vi "Test Tree Structure.vi"() -> ()   [LabVIEW 2014]
uses:
  ERP-Manage Work Orders/ERP-ManageWorkOrders.lvclass
panel:
  in  "Discard?":bool
  out "Navigate Tree:Get Parent Item 2":string
  out "Col 2":i32
  out "Tag":string
  out "String":string
  out "Navigate Tree:Get Child 2":string
  out "Array 2":string[](array[string])
  out "Navigate Tree:Get Parent Item":string
  out "Active Cell:String":string
  out "All Tags":string[](array[string])
  out "Navigate Tree:Get Child":string
  in  "Stop Button":bool
  out "Array":T1(array[cluster])
  in  "Tree":string(tree)
  in  "Data IN":string[][](array[string])
  in  "Items":T1(array[cluster])
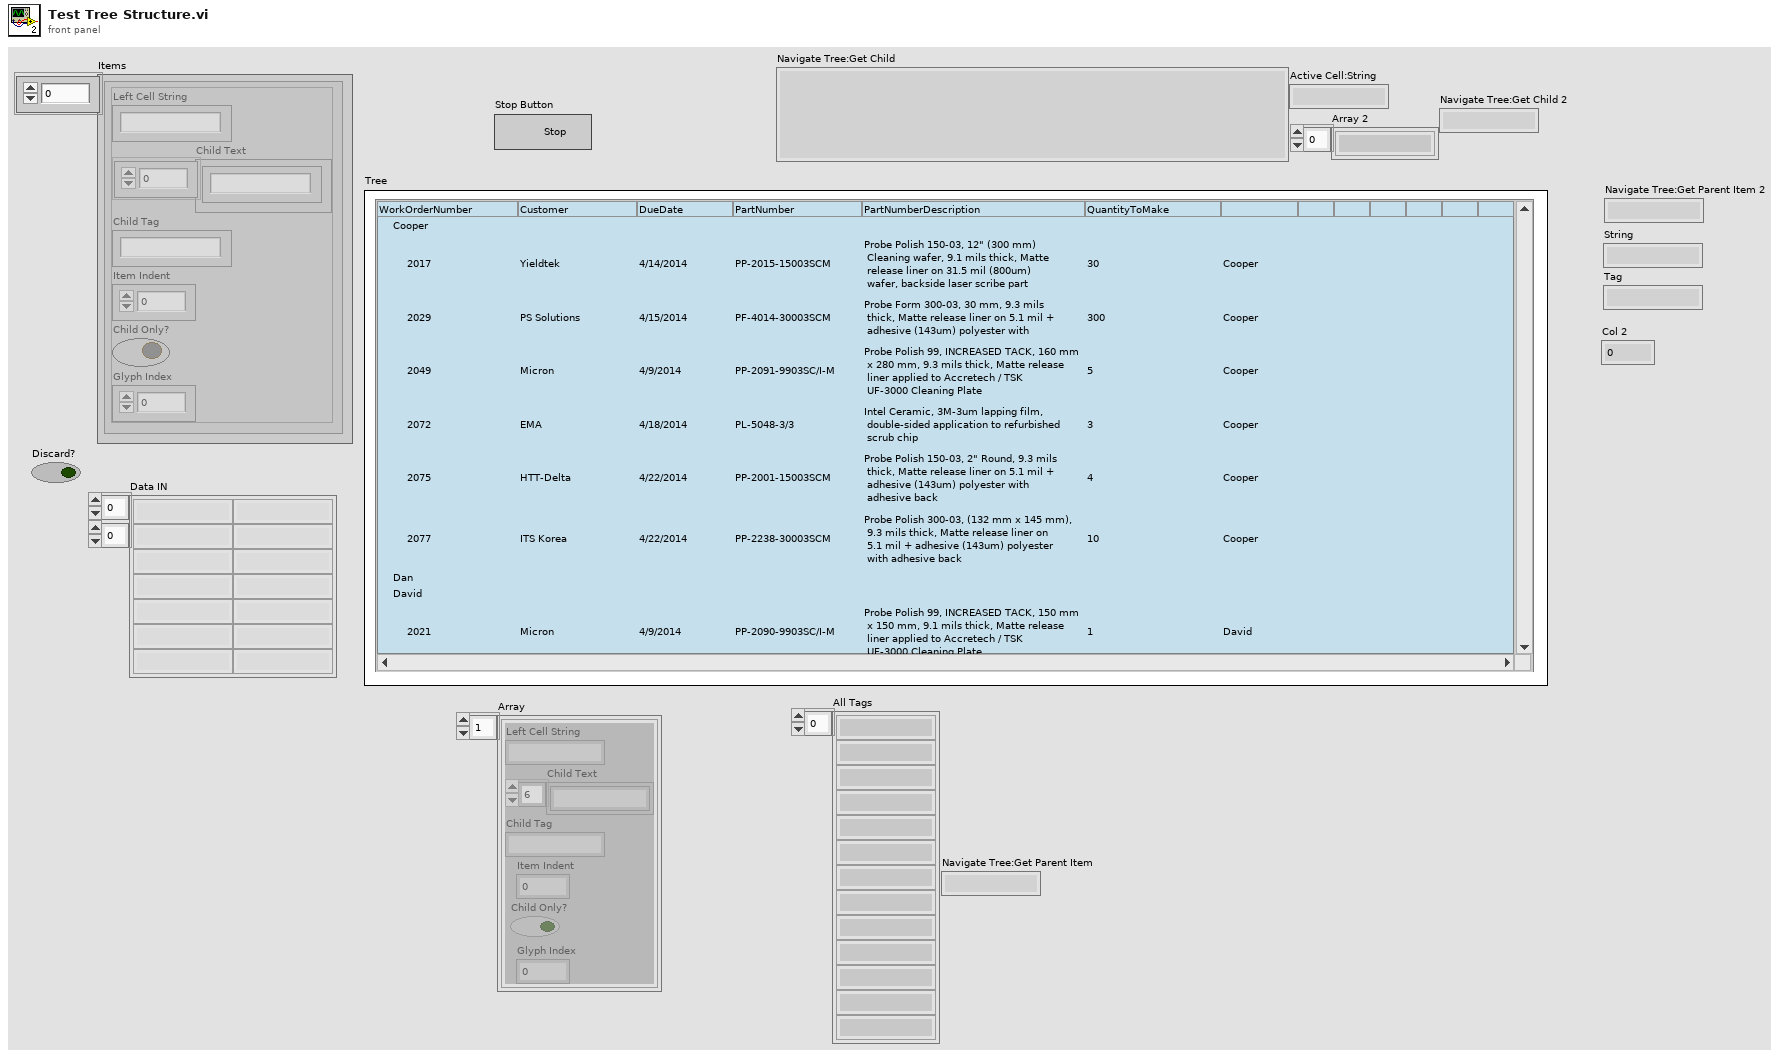
[diagram p1: front panel]
types:
  T1 = cluster{"Left Cell String":string, "Child Text":string[], "Child Tag":string, "Item Indent":i32, "Child Only?":bool, "Glyph Index":i32}[]
  T2 = cluster{"Left Cell String":string, "Child Text":string[], "Child Tag":string, "Item Indent":i32, "Child Only?":bool, "Glyph Index":i32}
  T3 = cluster{"data name":string, "drag data":variant}[]
  T4 = typedef "LVPoint32TypeDef.ctl" = cluster{"Horizontal":i32, "Vertical":i32}
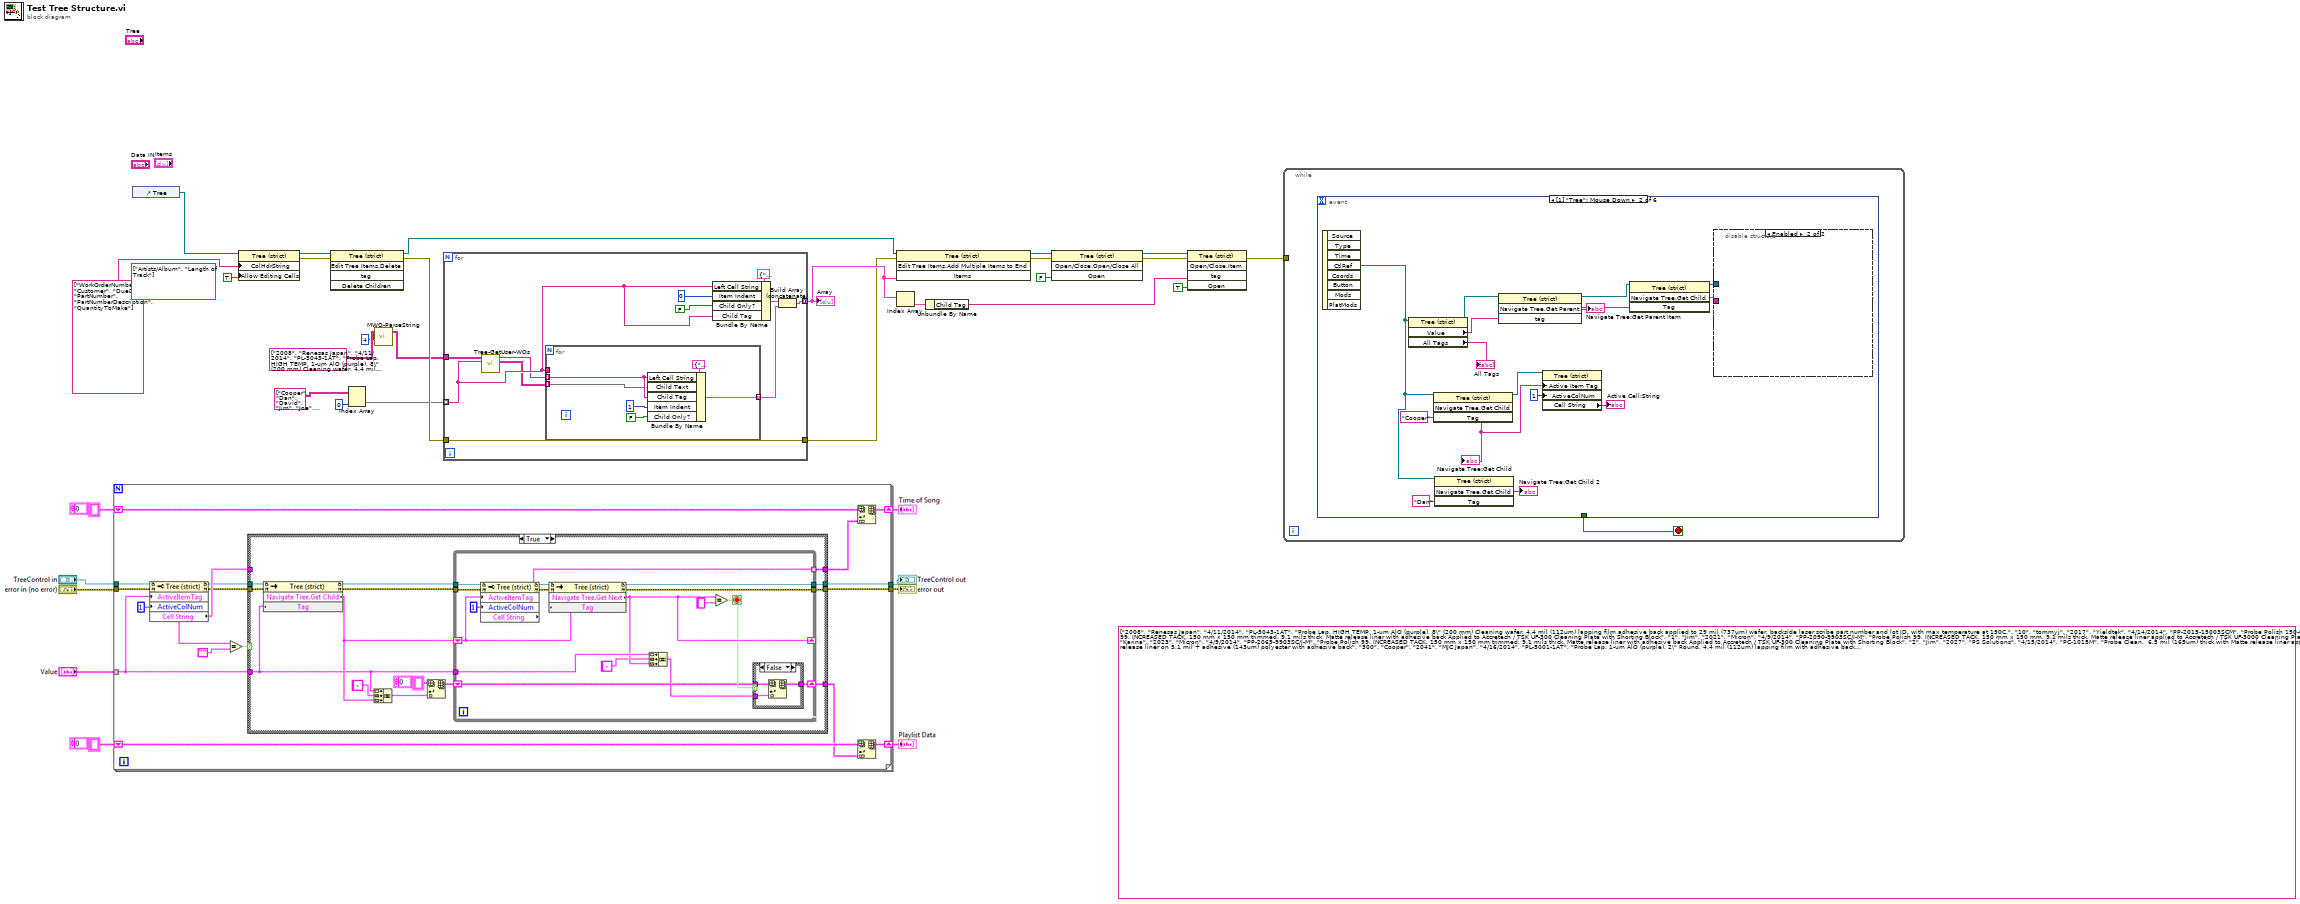
[diagram p0: block diagram]
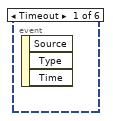
[diagram p2: hidden frame]
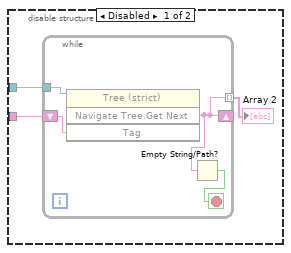
[diagram p3: hidden frame]
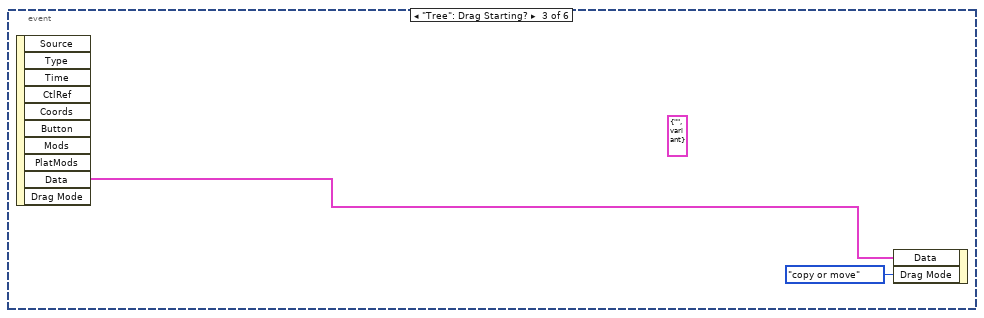
[diagram p4: hidden frame]
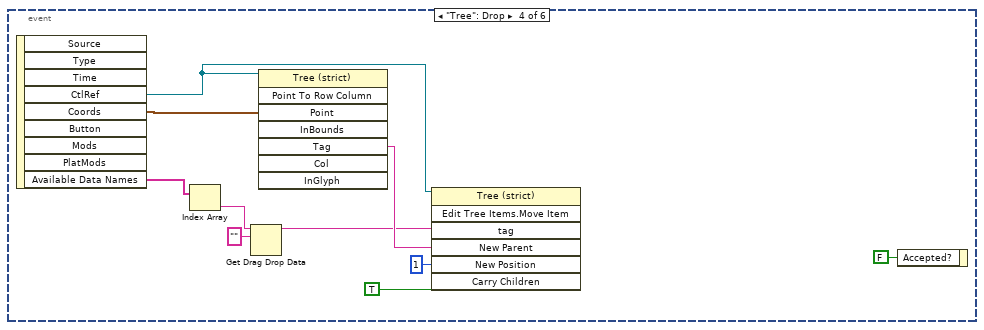
[diagram p5: hidden frame]
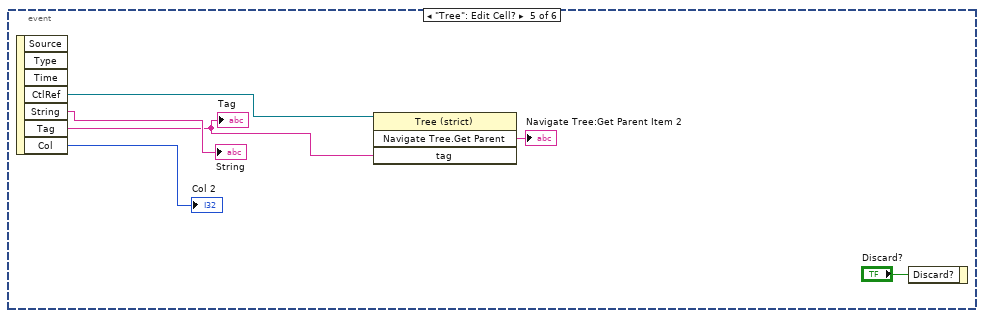
[diagram p6: hidden frame]
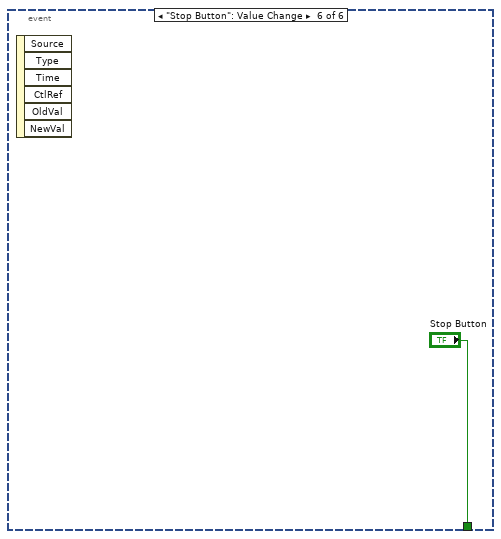
[diagram p7: hidden frame]
diagram:
  (unwired) string[][] [["2008", "Renesas Japan", "4/11/2014", "PL-5043-1AT", "Probe Lap, HIGH TEMP, 1-um AlO (purple), 8\" (200 mm) Cleaning wafer, 4.4 mil (112um) lapping film adhesive back applied to 29 mil (737um) wafer, backside laser scribe part number and lot ID. with max temperature at 150C.", "10", "tommyj"], ["2017", "Yieldtek", "4/14/2014", "PP-2015-15003SCM", "Probe Polish 150-03, 12\" (300 mm) Cleaning wafer, 9.1 mils thick, Matte release liner on 31.5 mil (800um) wafer, backside laser scribe part number and lot ID.", "30", "Cooper"], ["2018", "IM Flash", "4/11/2014", "PP-2069-9903SC/I-M", "Probe Polish 99, INCREASED TACK, 150 mm x 150 mm trimmed, 9.1 mils thick, Matte release liner with adhesive back Applied to Accretech / TSK UF-300 Cleaning Plate with Shorting Block", "1", "Jim"], ["2021", "Micron", "4/9/2014", "PP-2090-9903SC/I-M", "Probe Polish 99, INCREASED TACK, 150 mm x 150 mm, 9.1 mils thick, Matte release liner applied to Accretech / TSK UF-3000 Cleaning Plate", "1", "David"], ["2022", "Micron", "4/9/2014", "PP-2091-9903SC/I-M", "Probe Polish 99, INCREASED TACK, 160 mm x 280 mm, 9.3 mils thick, Matte release liner applied to Accretech / TSK UF-3000 Cleaning Plate", "5", "Karina"], ["2023", "Micron", "4/9/2014", "PP-2069-9903SC/I-M", "Probe Polish 99, INCREASED TACK, 150 mm x 150 mm trimmed, 9.1 mils thick, Matte release liner with adhesive back Applied to Accretech / TSK UF-300 Cleaning Plate with Shorting Block", "2", "Jim"], ["2027", "PS Solutions", "4/15/2014", "PC-1015M", "Probe Clean,  6.5 mil (165um) thick,with Matte release liner applied to 12\" (300 mm), 31.5 mil (800um) wafer, backside laser scribe part number and lot ID..", "2", "Karina"], ["2029", "PS Solutions", "4/15/2014", "PF-4014-30003SCM", "Probe Form 300-03, 30 mm, 9.3 mils thick, Matte release liner on 5.1 mil + adhesive (143um) polyester with adhesive back", "300", "Cooper"], ["2041", "MJC Japan", "4/16/2014", "PL-5001-1AT", "Probe Lap, 1-um AlO (purple), 2\" Round, 4.4 mil (112um) lapping film with adhesive back with max temperture at 150C", "87", "tommyj"], ["2047", "TeraProbe Japan", "4/16/2014", "PC-1012MX", "Probe Clean 8 inch cleaning wafer, 6.5 mils cleaning polymer with matte release liner on 29 mil (737um) wafer, backside laser scribe part number and lot ID.", "1", "Karina"], ["2048", "Micron", "4/9/2014", "PP-2090-9903SC/I-M", "Probe Polish 99, INCREASED TACK, 150 mm x 150 mm, 9.1 mils thick, Matte release liner applied to Accretech / TSK UF-3000 Cleaning Plate", "1", "David"], ["2049", "Micron", "4/9/2014", "PP-2091-9903SC/I-M", "Probe Polish 99, INCREASED TACK, 160 mm x 280 mm, 9.3 mils thick, Matte release liner applied to Accretech / TSK UF-3000 Cleaning Plate", "5", "Cooper"], ["2050", "Micron", "4/9/2014", "PP-2069-9903SC/I-M", "Probe Polish 99, INCREASED TACK, 150 mm x 150 mm trimmed, 9.1 mils thick, Matte release liner with adhesive back Applied to Accretech / TSK UF-300 Cleaning Plate with Shorting Block", "2", "Jim"], ["2053", "MJC Japan", "4/17/2014", "PP-2015-7003SCM-NEX", "Probe Polish 70, 12\" (300 mm) Cleaning wafer, 9.1 mils thick, Polished release liner applied to 31.5 mil (800um) wafer, backside laser scribe part number and lot ID. (No exclusion cut)", "1", "Jim"], ["2054", "MJC Japan", "4/17/2014", "PP-2015-7003SCM-NEX", "Probe Polish 70, 12\" (300 mm) Cleaning wafer, 9.1 mils thick, Polished release liner applied to 31.5 mil (800um) wafer, backside laser scribe part number and lot ID. (No exclusion cut)", "2", "tommyj"], ["2056", "Freescale ", "4/17/2014", "CCW-7043-01-150-FL", "Chuck Cleaning Wafer, 200 mm, 1.0X tack level, flat surface on 725 um wafer, backside laser scribe part number and lot ID, cleaning required for shipments to US, Japan, Europe, China, and Singapore. ", "1", "Rosey"], ["2108", "ITS Japan", "4/21/2014", "PP-2043-15003SCM", "Probe Polish 150-03, 8\" (200 mm) Cleaning wafer, 9.1 mils thick, Matte release liner applied to 29 mil (737um) wafer, backside laser scribe part number and lot ID.", "1", "David"], ["2111", "ITS Japan", "4/22/2014", "PL-5080-1AH", "Probe Lap, 1-um AlO (purple), 210 mm x 297 mm, 4.4 mil (112um) lapping film with adhesive back", "5", "Rosey"], ["2058", "Freescale", "4/17/2014", "PC-1043M", "Probe Clean, 8\" (200 mm) Cleaning wafer, 6.5 mil (165um) thick, Matte release liner applied to 29 mil (737um) wafer, backside laser scribe part number and lot ID.", "1", "tommyj"], ["2071", "Texas Instruments", "4/21/2014", "4700011-0001", "Probe Form 300-15, 1.5\" Square, 9.3 mils thick, Matte release liner on 5.1 mil + adhesive (143um) polyester with adhesive back", "35", "Rosey"], ["2072", "EMA", "4/18/2014", "PL-5048-3/3", "Intel Ceramic, 3M-3um lapping film, double-sided application to refurbished scrub chip", "3", "Cooper"], ["2073", "HTT-Melexis", "4/22/2014", "PP-2001-7003SCM", "Probe Polish 70, 2\" Round, 9.3 mils thick, Matte release liner on 5.1 mil + adhesive (143um) polyester with adhesive back..", "100", "Rosey"], ["2074", "HTT-Delta", "4/22/2014", "PP-2001-9903SC/I-M", "Probe Polish 99, 2\" Round, 9.3 mils thick, Matte release liner on 5.1 mil + adhesive (143um) polyester with adhesive back.", "4", "Jim"], ["2075", "HTT-Delta", "4/22/2014", "PP-2001-15003SCM", "Probe Polish 150-03, 2\" Round, 9.3 mils thick, Matte release liner on 5.1 mil + adhesive (143um) polyester with adhesive back", "4", "Cooper"], ["2076", "ITS Korea", "4/21/2014", "PC-1424M-O-B", "Probe Clean, 155 mm x 71 mm, 6.5 mils thick with 5 mil polyester, OPAQUE with matte release liner for CUSTOMER INSTALLATION", "38", "Rosey"], ["2077", "ITS Korea", "4/22/2014", "PP-2238-30003SCM", "Probe Polish 300-03, (132 mm x 145 mm), 9.3 mils thick, Matte release liner on 5.1 mil + adhesive (143um) polyester with adhesive back", "10", "Cooper"]] ("data")
  (unwired) string[] ["Artists/Album", "Length of Track"] ("Column Header Strings[]")
  n1 = control-ref of="Tree"() -> (w12:refnum<vi>)
  n2 = property on="Property Node" class="Tree (strict)"(reference=w12, "ColHdrString"=string[] ["WorkOrderNumber", "Customer", "DueDate", "PartNumber", "PartNumberDescription", "QuantityToMake"] ("columns"), "Allow Editing Cells"=TRUE) -> (reference out=w20:refnum<vi>, error out=w21:errorcluster)  [unwired: 1 in]
  n3 = invoke on="Invoke Node" class="Tree (strict)" method="Edit Tree Items.Delete"(reference=w20, error in=w21) -> (reference out=w19:refnum<vi>, error out=w9:errorcluster)  [unwired: 3 in, 3 out]
  n4 = Index Array(array=string[][] [["Cooper"], ["Dan"], ["David"], ["Jim"], ["Joe"], ["Kalynn"], ["Karina"], ["Mark"], ["Rosey"], ["tommyj"]] ("data"), index (col)=0 ("disabled index (col)")) -> (element=w8:string[])  [unwired: 1 in]
  n5 = call "MWO-ParseString.vi"("Work Order Data In"=string[][] [["2008", "Renesas Japan", "4/11/2014", "PL-5043-1AT", "Probe Lap, HIGH TEMP, 1-um AlO (purple), 8\" (200 mm) Cleaning wafer, 4.4 mil (112um) lapping film adhesive back applied to 29 mil (737um) wafer, backside laser scribe part number and lot ID. with max temperature at 150C.", "10", "tommyj"], ["2017", "Yieldtek", "4/14/2014", "PP-2015-15003SCM", "Probe Polish 150-03, 12\" (300 mm) Cleaning wafer, 9.1 mils thick, Matte release liner on 31.5 mil (800um) wafer, backside laser scribe part number and lot ID.", "30", "Cooper"], ["2018", "IM Flash", "4/11/2014", "PP-2069-9903SC/I-M", "Probe Polish 99, INCREASED TACK, 150 mm x 150 mm trimmed, 9.1 mils thick, Matte release liner with adhesive back Applied to Accretech / TSK UF-300 Cleaning Plate with Shorting Block", "1", "Jim"], ["2021", "Micron", "4/9/2014", "PP-2090-9903SC/I-M", "Probe Polish 99, INCREASED TACK, 150 mm x 150 mm, 9.1 mils thick, Matte release liner applied to Accretech / TSK UF-3000 Cleaning Plate", "1", "David"], ["2022", "Micron", "4/9/2014", "PP-2091-9903SC/I-M", "Probe Polish 99, INCREASED TACK, 160 mm x 280 mm, 9.3 mils thick, Matte release liner applied to Accretech / TSK UF-3000 Cleaning Plate", "5", "Karina"], ["2023", "Micron", "4/9/2014", "PP-2069-9903SC/I-M", "Probe Polish 99, INCREASED TACK, 150 mm x 150 mm trimmed, 9.1 mils thick, Matte release liner with adhesive back Applied to Accretech / TSK UF-300 Cleaning Plate with Shorting Block", "2", "Jim"], ["2027", "PS Solutions", "4/15/2014", "PC-1015M", "Probe Clean,  6.5 mil (165um) thick,with Matte release liner applied to 12\" (300 mm), 31.5 mil (800um) wafer, backside laser scribe part number and lot ID..", "2", "Karina"], ["2029", "PS Solutions", "4/15/2014", "PF-4014-30003SCM", "Probe Form 300-03, 30 mm, 9.3 mils thick, Matte release liner on 5.1 mil + adhesive (143um) polyester with adhesive back", "300", "Cooper"], ["2041", "MJC Japan", "4/16/2014", "PL-5001-1AT", "Probe Lap, 1-um AlO (purple), 2\" Round, 4.4 mil (112um) lapping film with adhesive back with max temperture at 150C", "87", "tommyj"], ["2047", "TeraProbe Japan", "4/16/2014", "PC-1012MX", "Probe Clean 8 inch cleaning wafer, 6.5 mils cleaning polymer with matte release liner on 29 mil (737um) wafer, backside laser scribe part number and lot ID.", "1", "Karina"], ["2048", "Micron", "4/9/2014", "PP-2090-9903SC/I-M", "Probe Polish 99, INCREASED TACK, 150 mm x 150 mm, 9.1 mils thick, Matte release liner applied to Accretech / TSK UF-3000 Cleaning Plate", "1", "David"], ["2049", "Micron", "4/9/2014", "PP-2091-9903SC/I-M", "Probe Polish 99, INCREASED TACK, 160 mm x 280 mm, 9.3 mils thick, Matte release liner applied to Accretech / TSK UF-3000 Cleaning Plate", "5", "Cooper"], ["2050", "Micron", "4/9/2014", "PP-2069-9903SC/I-M", "Probe Polish 99, INCREASED TACK, 150 mm x 150 mm trimmed, 9.1 mils thick, Matte release liner with adhesive back Applied to Accretech / TSK UF-300 Cleaning Plate with Shorting Block", "2", "Jim"], ["2053", "MJC Japan", "4/17/2014", "PP-2015-7003SCM-NEX", "Probe Polish 70, 12\" (300 mm) Cleaning wafer, 9.1 mils thick, Polished release liner applied to 31.5 mil (800um) wafer, backside laser scribe part number and lot ID. (No exclusion cut)", "1", "Jim"], ["2054", "MJC Japan", "4/17/2014", "PP-2015-7003SCM-NEX", "Probe Polish 70, 12\" (300 mm) Cleaning wafer, 9.1 mils thick, Polished release liner applied to 31.5 mil (800um) wafer, backside laser scribe part number and lot ID. (No exclusion cut)", "2", "tommyj"], ["2056", "Freescale ", "4/17/2014", "CCW-7043-01-150-FL", "Chuck Cleaning Wafer, 200 mm, 1.0X tack level, flat surface on 725 um wafer, backside laser scribe part number and lot ID, cleaning required for shipments to US, Japan, Europe, China, and Singapore. ", "1", "Rosey"], ["2108", "ITS Japan", "4/21/2014", "PP-2043-15003SCM", "Probe Polish 150-03, 8\" (200 mm) Cleaning wafer, 9.1 mils thick, Matte release liner applied to 29 mil (737um) wafer, backside laser scribe part number and lot ID.", "1", "David"], ["2111", "ITS Japan", "4/22/2014", "PL-5080-1AH", "Probe Lap, 1-um AlO (purple), 210 mm x 297 mm, 4.4 mil (112um) lapping film with adhesive back", "5", "Rosey"], ["2058", "Freescale", "4/17/2014", "PC-1043M", "Probe Clean, 8\" (200 mm) Cleaning wafer, 6.5 mil (165um) thick, Matte release liner applied to 29 mil (737um) wafer, backside laser scribe part number and lot ID.", "1", "tommyj"], ["2071", "Texas Instruments", "4/21/2014", "4700011-0001", "Probe Form 300-15, 1.5\" Square, 9.3 mils thick, Matte release liner on 5.1 mil + adhesive (143um) polyester with adhesive back", "35", "Rosey"], ["2072", "EMA", "4/18/2014", "PL-5048-3/3", "Intel Ceramic, 3M-3um lapping film, double-sided application to refurbished scrub chip", "3", "Cooper"], ["2073", "HTT-Melexis", "4/22/2014", "PP-2001-7003SCM", "Probe Polish 70, 2\" Round, 9.3 mils thick, Matte release liner on 5.1 mil + adhesive (143um) polyester with adhesive back..", "100", "Rosey"], ["2074", "HTT-Delta", "4/22/2014", "PP-2001-9903SC/I-M", "Probe Polish 99, 2\" Round, 9.3 mils thick, Matte release liner on 5.1 mil + adhesive (143um) polyester with adhesive back.", "4", "Jim"], ["2075", "HTT-Delta", "4/22/2014", "PP-2001-15003SCM", "Probe Polish 150-03, 2\" Round, 9.3 mils thick, Matte release liner on 5.1 mil + adhesive (143um) polyester with adhesive back", "4", "Cooper"], ["2076", "ITS Korea", "4/21/2014", "PC-1424M-O-B", "Probe Clean, 155 mm x 71 mm, 6.5 mils thick with 5 mil polyester, OPAQUE with matte release liner for CUSTOMER INSTALLATION", "38", "Rosey"], ["2077", "ITS Korea", "4/22/2014", "PP-2238-30003SCM", "Probe Polish 300-03, (132 mm x 145 mm), 9.3 mils thick, Matte release liner on 5.1 mil + adhesive (143um) polyester with adhesive back", "10", "Cooper"]] ("data"), "index (col)"=4) -> ("Work Order Data Out"=w2:string[][])  [unwired: 7 in]
  n6 = for {
    tunnel: [w30] -> w6 mode=concatenating
    tunnel: w9 -> [w29]
    tunnel: [w29] -> w5
    tunnel: w8 -> [w27] mode=indexing
    tunnel: w2 -> [w28]
    n7 = call "Tree-GetUser-WOs.vi"("User"=w27, "data"=w28) -> ("data out"=w26:string[][], "Work Orders"=w25:string[])  [unwired: 8 in]
    n8 = for {
      tunnel: [w40] -> w31 mode=indexing
      tunnel: w27 -> [_]
      tunnel: w25 -> [w37] mode=indexing
      tunnel: w26 -> [w36] mode=indexing
      n9 = Bundle By Name(cluster=T2 {"Left Cell String"="012914", "Child Text"=[], "Child Tag"="", "Item Indent"=0, "Child Only?"=FALSE, "Glyph Index"=0} ("Item"), "Left Cell String"=w37, "Child Text"=w36, "Child Tag"=w37, "Item Indent"=1, "Child Only?"=FALSE) -> (w40:T2)
    }
    n10 = Bundle By Name(cluster=T2 {"Left Cell String"="012914", "Child Text"=[], "Child Tag"="", "Item Indent"=0, "Child Only?"=FALSE, "Glyph Index"=0} ("Item"), "Left Cell String"=w27, "Item Indent"=0, "Child Only?"=FALSE, "Child Tag"=w27) -> (w32:T2)
    n11 = Build Array (concatenate)(w32, w31) -> (w30:T1)
  }
  "Array" <- w6
  n12 = invoke on="Invoke Node" class="Tree (strict)" method="Edit Tree Items.Add Multiple Items to End"(reference=w19, error in=w5, "Items"=w6) -> (reference out=w18:refnum<vi>, error out=w23:errorcluster)  [unwired: 1 in, 2 out]
  n13 = Index Array(array=w6) -> (element=w15:T2)  [unwired: 1 in]
  n14 = Unbundle By Name(w15) -> ("Child Tag"=w14:string)
  n15 = invoke on="Invoke Node" class="Tree (strict)" method="Open/Close.Open/Close All"(reference=w18, error in=w23, "Open"=FALSE ("Open?")) -> (reference out=w16:refnum<vi>, error out=w17:errorcluster)  [unwired: 1 in, 2 out]
  n16 = invoke on="Invoke Node" class="Tree (strict)" method="Open/Close.Item"(reference=w16, error in=w17, "tag"=w14, "Open"=TRUE ("Open?")) -> (error out=w4:errorcluster)  [unwired: 1 in, 4 out]
  n17 = while {
    tunnel: w4 -> [_]
    stop <- w42 stop-if-true
    n18 = event shown="[1] \"Tree\": Mouse Down" {
      selector: _ -> [_ _ _ _ _ _]
      dyn-events: _ -> [_ _ _ _ _ _]
      timeout: _ -> [_ _ _ _ _ _]
      tunnel: [_ _ _ _ _ "Stop Button"] -> w42
      event Timeout {
        n19 = event-data() -> ()  [unwired: 1 in, 3 out]
      }
      event "Tree": Mouse Down {
        n20 = event-data() -> ("CtlRef"=w44:refnum<vi>)  [unwired: 1 in, 7 out]
        n21 = property class="Tree (strict)"(reference=w44) -> (reference out=w50:refnum<vi>, "Value"=w51:string, "All Tags"=→"All Tags":string[])  [unwired: 1 in, 1 out]
        n22 = invoke class="Tree (strict)" method="Navigate Tree.Get Child"(reference=w44, "Tag"="Cooper") -> (reference out=w57:refnum<vi>, "Navigate Tree:Get Child"=w52:string)  [unwired: 2 in, 2 out]
        "Navigate Tree:Get Child" <- w52
        n23 = invoke class="Tree (strict)" method="Navigate Tree.Get Child"(reference=w44, "Tag"="Dan") -> ("Navigate Tree:Get Child"=→"Navigate Tree:Get Child 2":string)  [unwired: 2 in, 3 out]
        n24 = invoke class="Tree (strict)" method="Navigate Tree.Get Parent"(reference=w50, "tag"=w51) -> (reference out=w47:refnum<vi>, "Navigate Tree:Get Parent"=w49:string)  [unwired: 2 in, 2 out]
        "Navigate Tree:Get Parent Item" <- w49
        n25 = property class="Tree (strict)"(reference=w57, "Active Item Tag"=w52, "ActiveColNum"=1 ("Active Cell:Active Column Number")) -> ("Cell String"=→"Active Cell:String":string)  [unwired: 1 in, 2 out]
        n26 = invoke class="Tree (strict)" method="Navigate Tree.Get Child"(reference=w47, "Tag"=w49) -> (reference out=w46:refnum<vi>, "Navigate Tree:Get Child"=w48:string)  [unwired: 2 in, 2 out]
        n27 = disable-structure shown="Enabled" {
          disable-tunnel: w48 -> [w60 _]
          disable-tunnel: w46 -> [w59 _]
          frame Disabled {
            n28 = while {
              tunnel: w59 -> [w64]
              shift-right: [w61] -> _
              shift-left: w60 -> [w63]
              tunnel: [w61] -> w58 mode=indexing
              stop <- w62 stop-if-true
              n29 = invoke class="Tree (strict)" method="Navigate Tree.Get Next"(reference=w64, "Tag"=w63) -> ("Navigate Tree:Get Next Item"=w61:string)  [unwired: 2 in, 3 out]
              n30 = Empty String/Path?(string/path=w61) -> (empty?=w62:bool)
            }
            "Array 2" <- w58
          }
          frame Enabled {
          }
        }
      }
      event "Tree": Drag Starting? {
        (unwired) cluster{"data name":string, "drag data":variant} {"data name"="", "drag data"=variant}
        n31 = event-data() -> ("Data"=w65:T3)  [unwired: 1 in, 9 out]
        n32 = event-data("Data"=w65, "Drag Mode"=enum32{"copy or move", "copy only", "move only"}."copy or move") -> ()  [unwired: 1 in, 1 out]
      }
      event "Tree": Drop {
        n33 = event-data() -> ("CtlRef"=w74:refnum<vi>, "Coords"=w73:T4, "Available Data Names"=w76:string[])  [unwired: 1 in, 6 out]
        n34 = Index Array(array=w76) -> (element=w69:string)  [unwired: 1 in]
        n35 = Get Drag Drop Data(8:"" ("type"), 9:w69) -> (3:w67:string)  [unwired: 1 in, 1 out]
        n36 = invoke on="Invoke Node" class="Tree (strict)" method="Point To Row Column"(reference=w74, "Point"=w73) -> ("Tag"=w72:string)  [unwired: 6 in, 7 out]
        n37 = invoke on="Invoke Node" class="Tree (strict)" method="Edit Tree Items.Move Item"(reference=w74, "tag"=w67, "New Parent"=w72, "New Position"=1, "Carry Children"=TRUE ("Carry Children?")) -> ()  [unwired: 2 in, 7 out]
        n38 = event-data("Accepted?"=FALSE) -> ()  [unwired: 1 in, 1 out]
      }
      event "Tree": Edit Cell? {
        n39 = event-data() -> ("CtlRef"=w81:refnum<vi>, "String"=→"String":string, "Tag"=w78:string, "Col"=→"Col 2":i32)  [unwired: 1 in, 3 out]
        "Tag" <- w78
        n40 = invoke on="Invoke Node" class="Tree (strict)" method="Navigate Tree.Get Parent"(reference=w81, "tag"=w78) -> ("Navigate Tree:Get Parent"=→"Navigate Tree:Get Parent Item 2":string)  [unwired: 2 in, 3 out]
        n41 = event-data("Discard?"="Discard?") -> ()  [unwired: 1 in, 1 out]
      }
      event "Stop Button": Value Change {
        n42 = event-data() -> ()  [unwired: 1 in, 6 out]
      }
    }
  }
